vi "SeCrTs-NS Send to RD Data.vi"(10 "Data FIFO Ref":T1) -> (3 "Cluster":T2)   [LabVIEW 2022 SP3]
uses:
  RT Controls/Data FIFO.ctl
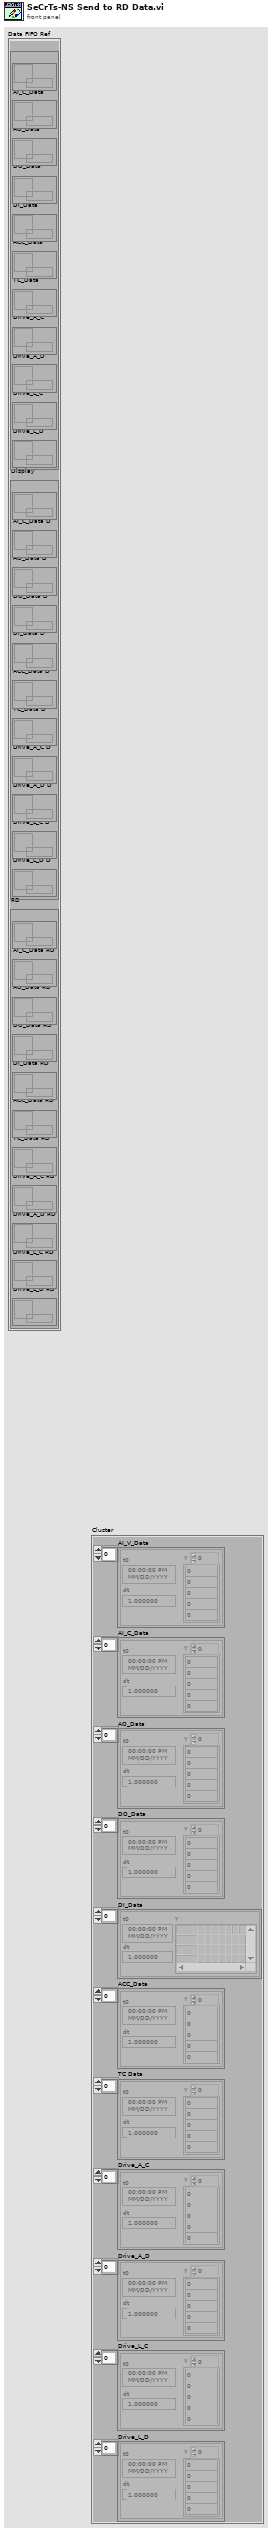
[diagram p1: front panel]
types:
  T1 = typedef "Data FIFO.ctl" = cluster{"Control":cluster{"AI_V_Data":refnum<queue>, "AI_C_Data":refnum<queue>, "AO_Data":refnum<queue>, "DO_Data":refnum<queue>, "DI_Data":refnum<queue>, "ACC_Data":refnum<queue>, "TC_Data":refnum<queue>, "Drive_A_C":refnum<queue>, "Drive_A_D":refnum<queue>, "Drive_L_C":refnum<queue>, "Drive_L_D":refnum<queue>}, "Display":cluster{"AI_V_Data D":refnum<queue>, "AI_C_Data D":refnum<queue>, "AO_Data D":refnum<queue>, "DO_Data D":refnum<queue>, "DI_Data D":refnum<queue>, "ACC_Data D":refnum<queue>, "TC_Data D":refnum<queue>, "Drive_A_C D":refnum<queue>, "Drive_A_D D":refnum<queue>, "Drive_L_C D":refnum<queue>, "Drive_L_D D":refnum<queue>}, "RD":cluster{"AI_V_Data RD":refnum<queue>, "AI_C_Data RD":refnum<queue>, "AO_Data RD":refnum<queue>, "DO_Data RD":refnum<queue>, "DI_Data RD":refnum<queue>, "ACC_Data RD":refnum<queue>, "TC_Data RD":refnum<queue>, "Drive_A_C RD":refnum<queue>, "Drive_A_D RD":refnum<queue>, "Drive_L_C RD":refnum<queue>, "Drive_L_D RD":refnum<queue>}}
  T2 = cluster{"AI_V_Data":waveform(dbl)[], "AI_C_Data":waveform(dbl)[], "AO_Data":waveform(dbl)[], "DO_Data":waveform(dbl)[], "DI_Data":digitalwaveform[], "ACC_Data":waveform(dbl)[], "TC Data":waveform(dbl)[], "Drive_A_C":waveform(dbl)[], "Drive_A_D":waveform(dbl)[], "Drive_L_C":waveform(dbl)[], "Drive_L_D":waveform(dbl)[]}
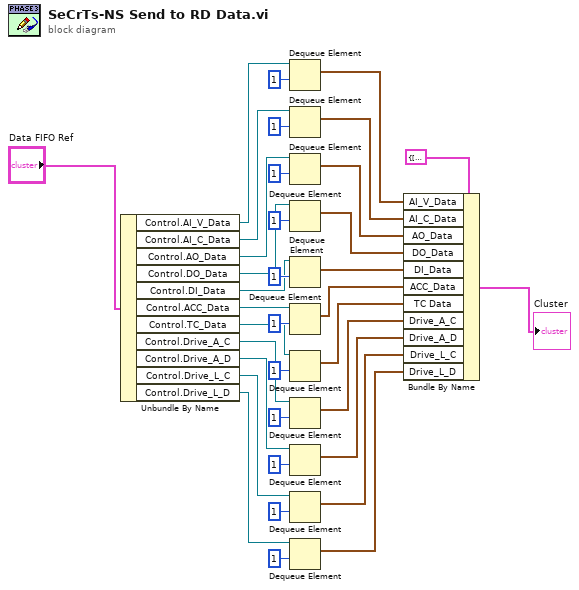
[diagram p0: block diagram]
diagram:
  n1 = Unbundle By Name("Data FIFO Ref") -> ("Control.AI_V_Data"=w2:refnum<queue>, "Control.AI_C_Data"=w3:refnum<queue>, "Control.AO_Data"=w4:refnum<queue>, "Control.DO_Data"=w5:refnum<queue>, "Control.DI_Data"=w6:refnum<queue>, "Control.ACC_Data"=w7:refnum<queue>, "Control.TC_Data"=w8:refnum<queue>, "Control.Drive_A_C"=w9:refnum<queue>, "Control.Drive_A_D"=w10:refnum<queue>, "Control.Drive_L_C"=w11:refnum<queue>, "Control.Drive_L_D"=w12:refnum<queue>)
  n2 = Dequeue Element(queue=w2, timeout in ms (-1)=1) -> (element=w13:waveform(dbl)[])  [unwired: 1 in, 3 out]
  n3 = Dequeue Element(queue=w3, timeout in ms (-1)=1) -> (element=w22:waveform(dbl)[])  [unwired: 1 in, 3 out]
  n4 = Dequeue Element(queue=w4, timeout in ms (-1)=1) -> (element=w14:waveform(dbl)[])  [unwired: 1 in, 3 out]
  n5 = Dequeue Element(queue=w5, timeout in ms (-1)=1) -> (element=w15:waveform(dbl)[])  [unwired: 1 in, 3 out]
  n6 = Dequeue Element(queue=w6, timeout in ms (-1)=1) -> (element=w16:digitalwaveform[])  [unwired: 1 in, 3 out]
  n7 = Dequeue Element(queue=w7, timeout in ms (-1)=1) -> (element=w17:waveform(dbl)[])  [unwired: 1 in, 3 out]
  n8 = Dequeue Element(queue=w8, timeout in ms (-1)=1) -> (element=w18:waveform(dbl)[])  [unwired: 1 in, 3 out]
  n9 = Dequeue Element(queue=w9, timeout in ms (-1)=1) -> (element=w19:waveform(dbl)[])  [unwired: 1 in, 3 out]
  n10 = Dequeue Element(queue=w10, timeout in ms (-1)=1) -> (element=w20:waveform(dbl)[])  [unwired: 1 in, 3 out]
  n11 = Dequeue Element(queue=w11, timeout in ms (-1)=1) -> (element=w21:waveform(dbl)[])  [unwired: 1 in, 3 out]
  n12 = Dequeue Element(queue=w12, timeout in ms (-1)=1) -> (element=w24:waveform(dbl)[])  [unwired: 1 in, 3 out]
  n13 = Bundle By Name(cluster=T2 {"AI_V_Data"=[], "AI_C_Data"=[], "AO_Data"=[], "DO_Data"=[], "DI_Data"=[], "ACC_Data"=[], "TC Data"=[], "Drive_A_C"=[], "Drive_A_D"=[], "Drive_L_C"=[], "Drive_L_D"=[]}, "AI_V_Data"=w13, "AI_C_Data"=w22, "AO_Data"=w14, "DO_Data"=w15, "DI_Data"=w16, "ACC_Data"=w17, "TC Data"=w18, "Drive_A_C"=w19, "Drive_A_D"=w20, "Drive_L_C"=w21, "Drive_L_D"=w24) -> (→"Cluster":T2)
